vi "main.vi"(8 "Error in":errorcluster) -> (0 "Error out":errorcluster)   [LabVIEW 2018, in "Error Handler.lvlib"]
uses:
  Error Handler.lvlib
  Common/Common.lvlib
  ctl/Module Queue - Action.ctl
  ctl/Module - State.ctl
  Common/ctl/Stop All - Action.ctl
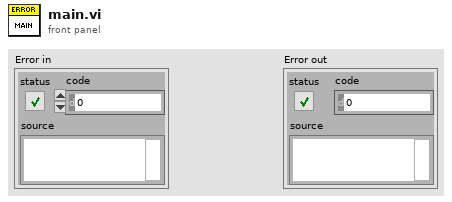
[diagram p1: front panel]
types:
  T1 = typedef "Error Handler.lvlib/Module Queue - Action.ctl" = enum16{"Create", "Get", "Destroy"}
  T2 = typedef "Common.lvlib/Stop All - Action.ctl" = enum16{"Create", "Fire", "Get", "Destroy"}
  T3 = typedef "Error Handler.lvlib/Module - State.ctl" = enum16{"Init", "Idle", "Error", "Close", "Handle External Error", "Log Error"}
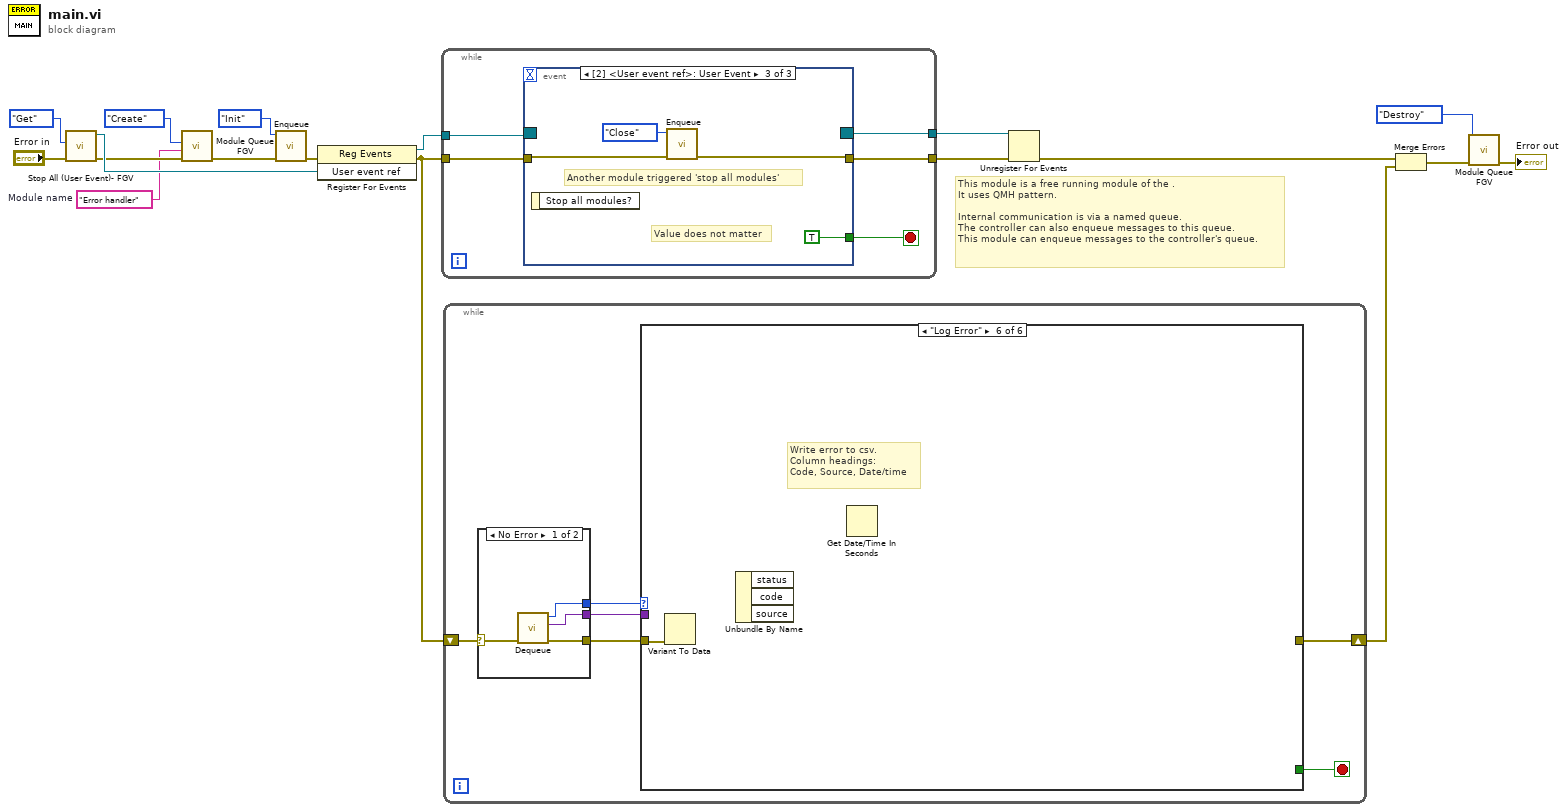
[diagram p0: block diagram]
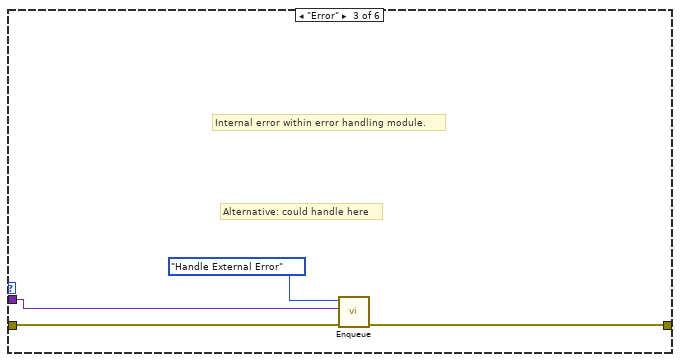
[diagram p4: hidden frame]
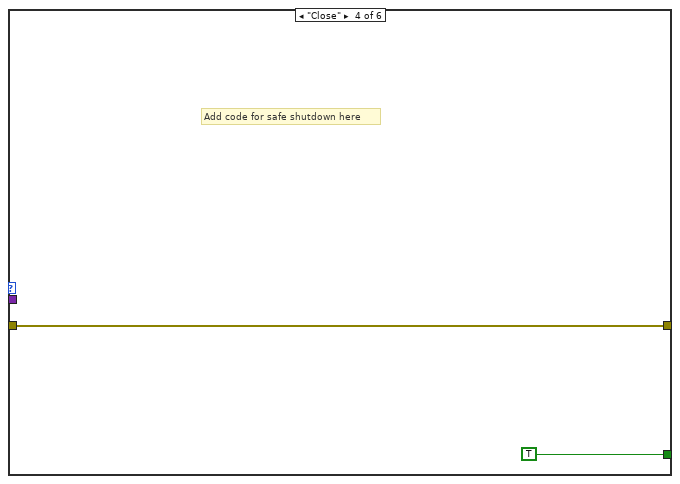
[diagram p5: hidden frame]
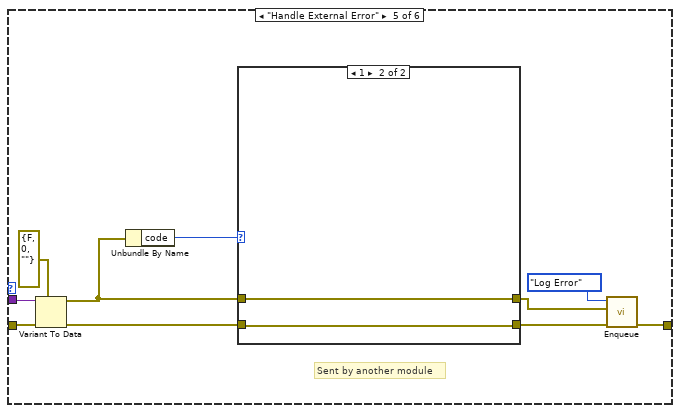
[diagram p6: hidden frame]
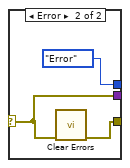
[diagram p8: hidden frame]
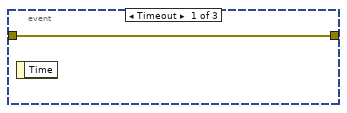
[diagram p9: hidden frame]
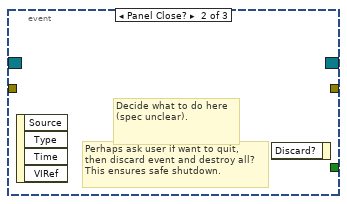
[diagram p10: hidden frame]
diagram:
  w1 = "Error handler"  # Module name
  # "This module is a free running module of the .\nIt uses QMH pattern.\n\nInternal communication is via a named queue.\nThe controller can also enqueue messages to this queue.\nThis module can enqueue messages to the controller's queue."
  n1 = call "Stop All (User Event)- FGV.vi"("error in"="Error in", "Action"=Stop_All_-_Action."Get") -> ("error out"=w9:errorcluster, "User event ref"=w14:refnum<user-event>)  [unwired: 8 in]
  n2 = call "Module Queue FGV.vi"("Error in"=w9, "Queue name"=w1, "Action"=Module_Queue_-_Action."Create") -> ("Error out"=w17:errorcluster)  [unwired: 7 in, 1 out]
  n3 = call "Enqueue.vi"("error in (no error)"=w17, "State"=Module_-_State."Init") -> ("error out"=w8:errorcluster)  [unwired: 9 in]
  n4 = register-events(error in=w8, w14) -> (reference out=w12:refnum<event-registration>, error out=w3:errorcluster)  [unwired: 1 in]
  n5 = while {
    tunnel: w12 -> [w23]
    tunnel: [w22] -> w11
    tunnel: w3 -> [w21]
    tunnel: [w20] -> w10
    stop <- w19 stop-if-true
    n6 = event shown="[2] <User event ref>: User Event" {
      selector: w23 -> [_ _ _]
      dyn-events: [_ _ _] -> w22
      timeout: _ -> [_ _ _]
      tunnel: w21 -> [w24 _ w28]
      tunnel: [w24 _ w27] -> w20
      tunnel: [_ _ TRUE] -> w19
      event Timeout {
        n7 = event-data() -> ()  [unwired: 1 in, 1 out]
      }
      event Panel Close? {
        # "Perhaps ask user if want to quit,\nthen discard event and destroy all?\nThis ensures safe shutdown."
        # "Decide what to do here\n(spec unclear)."
        n8 = event-data() -> ()  [unwired: 1 in, 4 out]
        n9 = event-data() -> ()  [unwired: 2 in, 1 out]
      }
      event User Event {
        # "Value does not matter"
        # "Another module triggered 'stop all modules'"
        n10 = event-data() -> ()  [unwired: 1 in, 1 out]
        n11 = call "Enqueue.vi"("error in (no error)"=w28, "State"=Module_-_State."Close") -> ("error out"=w27:errorcluster)  [unwired: 9 in]
      }
    }
  }
  n12 = while {
    shift-right: [w29] -> w2
    shift-left: w3 -> [w34]
    stop <- w30 stop-if-true
    n13 = case shown="No Error" w34 {
      selector: w34 -> [w58 w60]
      tunnel: [w57 Module_-_State."Error" ("State")] -> w33
      tunnel: [w56 w60] -> w32
      tunnel: [w55 w59] -> w31
      frame No Error {
        n14 = call "Dequeue.vi"("error in"=w58) -> ("error out"=w55:errorcluster, "Data"=w56:variant, "State"=w57:T3)  [unwired: 8 in]
      }
      frame Error {
        # "Instead of dequeue,\nhandle the error"
        n15 = call <vilib>:"Clear Errors.vi"("error in (no error)"=w60) -> ("error out"=w59:errorcluster)  [unwired: 5 in, 1 out]
      }
    }
    n16 = case shown="\"Log Error\"" w33 {
      tunnel: w32 -> [_ _ w36 _ w50 _]
      tunnel: w31 -> [_ w35 w38 w40 w51 w54]
      tunnel: [_ _ _ TRUE _ _] -> w30
      tunnel: [_ w35 w37 w40 w42 _] -> w29
      frame "Init", Default {
      }
      frame "Idle" {
      }
      frame "Error" {
        # "Alternative: could handle here"
        # "Internal error within error handling module."
        n17 = call "Enqueue.vi"("error in (no error)"=w38, "Data"=w36, "State"=Module_-_State."Handle External Error") -> ("error out"=w37:errorcluster)  [unwired: 8 in]
      }
      frame "Close" {
        # "Add code for safe shutdown here"
      }
      frame "Handle External Error" {
        # "Sent by another module"
        n18 = Variant To Data(error in=w51, type=errorcluster {"status"=FALSE, "code"=0, "source"=""} ("error constant"), Variant=w50) -> (data=w44:errorcluster, error out=w47:errorcluster)
        n19 = Unbundle By Name(w44) -> ("code"=w48:i32)
        n20 = case shown="1" w48 {
          tunnel: [_ w53] -> w43
          tunnel: w47 -> [_ w53]
          tunnel: [_ w52] -> w45
          tunnel: w44 -> [_ w52]
          frame 0, Default {
          }
          frame 1 {
          }
        }
        n21 = call "Enqueue.vi"("error in (no error)"=w43, "Data"=w45, "State"=Module_-_State."Log Error") -> ("error out"=w42:errorcluster)  [unwired: 8 in]
      }
      frame "Log Error" {
        # "Write error to csv.\nColumn headings:\nCode, Source, Date/time"
        n22 = Variant To Data(error in=w54) -> ()  [unwired: 2 in, 2 out]
        n23 = Unbundle By Name() -> ()  [unwired: 1 in, 3 out]
        n24 = Get Date/Time In Seconds() -> ()  [unwired: 1 out]
      }
    }
  }
  n25 = Unregister For Events(event registration refnum=w11, error in=w10) -> (error out=w7:errorcluster)
  n26 = Merge Errors(w7, w2) -> (w6:errorcluster)
  n27 = call "Module Queue FGV.vi"("Error in"=w6, "Action"=Module_Queue_-_Action."Destroy") -> ("Error out"=→"Error out":errorcluster)  [unwired: 8 in, 1 out]
